vi "test_float.vi"() -> ()   [LabVIEW 2018]
panel:
  out "*(type *) &x":u8[](array[numeric]) format="%x"
  in  "Numeric":sgl
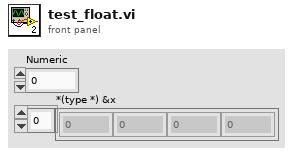
[diagram p1: front panel]
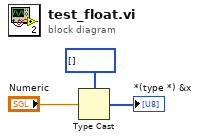
[diagram p0: block diagram]
diagram:
  n1 = Type Cast(type=u8[] [], x="Numeric") -> (*(type *) &x=→"*(type *) &x":u8[])
